vi "Layout - Load Layout-VI Reference.vi"(8 "error in (no error)":errorcluster, 11 "hse-config":refnum<class "config-base.lvclass">) -> (0 "error out":errorcluster, 3 "Layout-VI Ref":refnum<vi>)   [LabVIEW 2022 SP3, in "UI Manager.lvlib"]
doc: "Opens the VI reference to the layout VI (the VI holding the panes and subpanels for the actual module display). \n\n____\nHAMPEL SOFTWARE ENGINEERING v2.6.0 (2023-12-19 10:54)"
uses:
  UI Manager.lvlib
  Libraries/hse-libraries/Source/hse-configuration/config-base/config-base.lvclass
  Project/PROJECT_Layout-VI.vi
  Libraries/hse-libraries/Source/hse-application/hse-application.lvclass
  Project/Project.lvlib
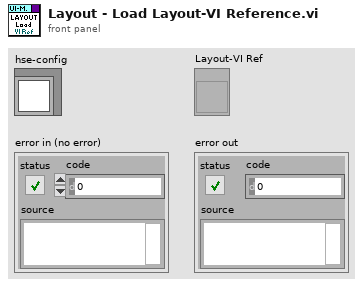
[diagram p1: front panel]
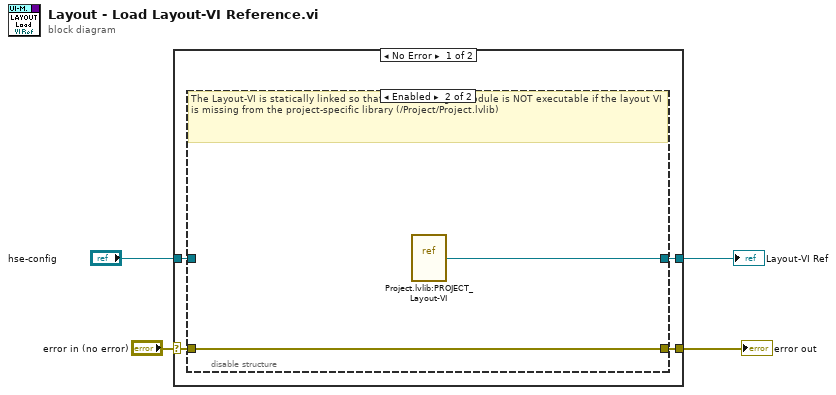
[diagram p0: block diagram]
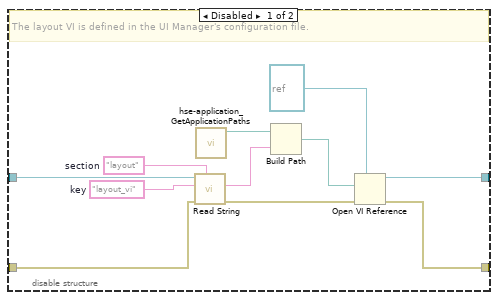
[diagram p2: hidden frame]
diagram:
  n1 = case shown="No Error" "error in (no error)" {
    selector: "error in (no error)" -> [w6 w22]
    tunnel: [w8 _] -> w3
    tunnel: "hse-config" -> [w7 _]
    tunnel: [w5 w22] -> w1
    frame No Error {
      n2 = disable-structure shown="Enabled" {
        disable-tunnel: [w17 w21] -> w8
        disable-tunnel: w7 -> [w16 _]
        disable-tunnel: w6 -> [w12 w20]
        disable-tunnel: [w10 w20] -> w5
        frame Disabled {
          w15 = "layout_vi"  # key
          w9 = "layout"  # section
          # "The layout VI is defined in the UI Manager's configuration file."
          n3 = call-dynamic "Read String.vi"("Section"=w9, "error in"=w12, "Key"=w15, "config-base in"=w16) -> ("error out"=w11:errorcluster, "Value"=w14:string)  [unwired: 5 in, 1 out]
          n4 = call "hse-application_GetApplicationPaths.vi"() -> ("Application Directory"=w13:path)  [unwired: 5 in, 6 out]
          n5 = Build Path(base path=w13, name or relative path=w14) -> (appended path=w18:path)
          n6 = Open VI Reference(type specifier VI Refnum (for type only)=refnum<vi> refnum, vi path=w18, error in (no error)=w11) -> (vi reference=w17:refnum<vi>, error out=w10:errorcluster)  [unwired: 3 in]
        }
        frame Enabled {
          # "The Layout-VI is statically linked so that the UI Manager module is NOT executable if the layout VI is missing from the project-specific library (/Project/Project.lvlib)"
          n7 = vi-ref "Project.lvlib:PROJECT_Layout-VI.vi"() -> (w21:refnum<vi>)
        }
      }
    }
    frame Error {
    }
  }
  "error out" <- w1
  "Layout-VI Ref" <- w3
